vi "Generate Control UI control refs file.vi"() -> ()   [LabVIEW 2017]
uses:
  <vilib>/TELLC/CtrlRef/TD UI Control Label-IONames--cluster.ctl
  <vilib>/TELLC/CtrlRef/TD UI Control Label-Alias-IOName--cluster.ctl
  <vilib>/TELLC/CtrlRef/TD Control refs--cluster.ctl
  <userlib>/_OpenG.lib/appcontrol/appcontrol.llb/ClassID Names Enum__ogtk.ctl
panel:
  in  "UI vi absolute path":path=path "C:/Projects/Ichor/AVC2/LV_Source/Application/AVC2_TouchScreen_MainUI.vi"
  out "Size":i32
  out "error out":errorcluster
  in  "ConfigFile":path
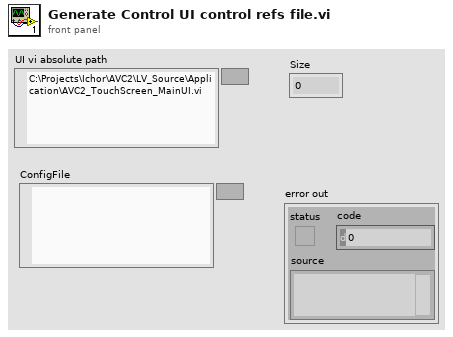
[diagram p1: front panel]
types:
  T1 = typedef "TD UI Control Label-IONames--cluster.ctl" = cluster{"Controls":T2[]}
  T2 = typedef "TD UI Control Label-Alias-IOName--cluster.ctl" = cluster{"Label":string, "Alias":string, "IOName":string}
  T3 = typedef "TD Control refs--cluster.ctl" = cluster{"label":string, "ClassID Name":T4, "ref":refnum<vi>, "Alias":string, "IOName":string}
  T4 = typedef "ClassID Names Enum__ogtk.ctl" = enum32{"0 <undefined>", "1 <undefined>", "2 <undefined>", "Generic", "Decoration", "Text", "Control", "ColorBox", "Boolean", "RefNum", "Variant", "Path", "ListBox", "Table", "Array", "Picture", "ActiveXContainer", "Numeric", "Digital", "NamedNumeric", "ColorRamp", "Slide", "GraphOrChart", "WaveformChart", "WaveformGraph", "IntensityChart", "IntensityGraph", "String", "IOName", "ComboBox", "Cluster", "Panel", "Knob", "NumWithScale", "Ring", "Enum", "GObject", "Plot", "Cursor", "NumericText", "Scale", "ColorScale", "GraphScale", "ColorGraphScale", "TypedRefNum", "OldKnobScale", "MCListbox", "MeasureData", "BVTag", "DAQName", "VISAName", "IVIName", "SlideScale", "TabControl", "Page", "TabArrayTabControl", "ConPane"}
  T5 = cluster{"Label":string, "ClassID Name":T4, "CtrlRef":refnum<vi>}[]
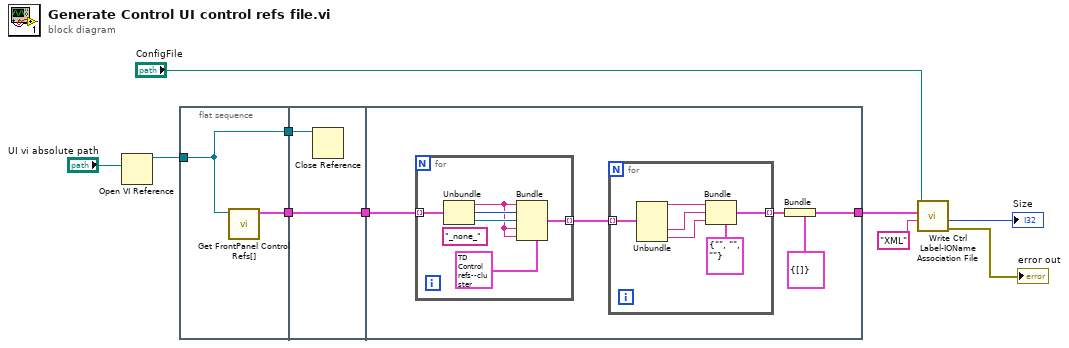
[diagram p0: block diagram]
diagram:
  n1 = Open VI Reference(vi path="UI vi absolute path") -> (vi reference=w10:refnum<vi>)  [unwired: 5 in, 1 out]
  n2 = flat-sequence {
    tunnel: w10 -> [w11]
    tunnel: [w12] -> w3
    tunnel: [w11] -> w1
    tunnel: w3 -> [w14]
    tunnel: [w14] -> w2
    tunnel: w1 -> [w13]
    tunnel: w2 -> [w19]
    tunnel: [w15] -> w8
    frame #0 {
      n3 = call <vilib>:"Get FrontPanel Control Refs[].vi"("VI (Caller)"=w11) -> ("ControlRefs[]"=w12:T5)  [unwired: 8 in, 2 out]
    }
    frame #1 {
      n4 = Close Reference(reference=w13) -> ()  [unwired: 1 in, 1 out]
    }
    frame #2 {
      n5 = for {
        tunnel: w19 -> [w28] mode=indexing
        tunnel: [w26] -> w18 mode=indexing
        (unwired) "_none_"
        n6 = Unbundle(w28) -> ("Label"=w27:string, "ClassID Name"=w31:T4, "CtrlRef"=w30:refnum<vi>)
        n7 = Bundle(cluster=T3 {"label"="", "ClassID Name"=enum."0 <undefined>", "ref"=refnum, "Alias"="", "IOName"=""} ("control refs"), "label"=w27, "ClassID Name"=w31, "ref"=w30, "Alias"=w27, "IOName"=w27) -> (w26:T3)
      }
      n8 = for {
        tunnel: w18 -> [w25] mode=indexing
        tunnel: [w20] -> w16 mode=indexing
        n9 = Unbundle(w25) -> ("label"=w24:string, "Alias"=w23:string, "IOName"=w22:string)  [unwired: 2 out]
        n10 = Bundle(cluster=T2 {"Label"="", "Alias"="", "IOName"=""} ("Label Associations"), "Label"=w24, "Alias"=w23, "IOName"=w22) -> (w20:T2)
      }
      n11 = Bundle(cluster=T1 {"Controls"=[]} ("UI Control Label Associations"), "Controls"=w16) -> (w15:T1)
    }
  }
  n12 = call <vilib>:"Write Ctrl Label-IOName Association File.vi"("file extension"="XML", "UI Control Label Associations"=w8, "ConfigFile"="ConfigFile") -> ("error out"=→"error out":errorcluster, "Size"=→"Size":i32)  [unwired: 7 in]
